vi "calc T and P.vi"(7 "DAQ state cluster in in":T1={"DAQ state"=enum."Global comm", "device"="", "start (ms)"=0, "error"={"status"=FALSE, "code"=0, "source"=""}, "T cont"={"exec"={"T mode"=enum."Setting up", "man power"=0.0, "log"=FALSE}, "T status"={"Temp"=0.0, "Power"=0.0}, "utility"={"meas index"=0, "wait (ms)"=0, "H Vmax"=8.5, "power out"=5.0, "heat volt out"=0.0, "heat volt in"=0.0, "therm volt"=0.0, "t T P hist"=[]}}} {"T cont"."utility"."therm volt" format="%_6g"; "T cont"."utility"."heat volt in" format="%_6g"; "T cont"."utility"."heat volt out" format="%_6g"; "T cont"."utility"."power out" format="%_6g"; "T cont"."utility"."H Vmax" format="%_6g"; "T cont"."exec"."man power" format="%_6g"; "T cont"."T status"."Power" format="%_6g"; "T cont"."T status"."Temp" format="%_6g"}) -> (8 "DAQ state cluster out":T1={"DAQ state"=enum."Global comm", "device"="", "start (ms)"=0, "error"={"status"=FALSE, "code"=0, "source"=""}, "T cont"={"exec"={"T mode"=enum."Setting up", "man power"=0.0, "log"=FALSE}, "T status"={"Temp"=0.0, "Power"=0.0}, "utility"={"meas index"=0, "wait (ms)"=0, "H Vmax"=8.5, "power out"=5.0, "heat volt out"=0.0, "heat volt in"=0.0, "therm volt"=0.0, "t T P hist"=[]}}} {"T cont"."utility"."therm volt" format="%_6g"; "T cont"."utility"."heat volt in" format="%_6g"; "T cont"."utility"."heat volt out" format="%_6g"; "T cont"."utility"."power out" format="%_6g"; "T cont"."utility"."H Vmax" format="%_6g"; "T cont"."exec"."man power" format="%_6g"; "T cont"."T status"."Power" format="%_6g"; "T cont"."T status"."Temp" format="%_6g"})   [LabVIEW 2019]
doc: "This subVI is a component of the meas T and P state of the DAQ state machine in the bug experiment.\n\nThis subVI calculates the current time, the bug temerature, and the bug heater power from the raw voltage measurements and saves the data to arunning array for graphing.\n\nIt records the history of the time, temperature, and power.\nIt also logs the temp control parameters is logging is active.\n\nPaul K Dixon\nP3600\nCSUSB Physics"
uses:
  typedefs/DAQ T state cluster.ctl
  typedefs/DAQ T state enum.ctl
  typedefs/temp cont cluster.ctl
  typedefs/temp exec cluster.ctl
  typedefs/temp mode enum.ctl
  typedefs/temp indicator.ctl
  typedefs/temp cont utility.ctl
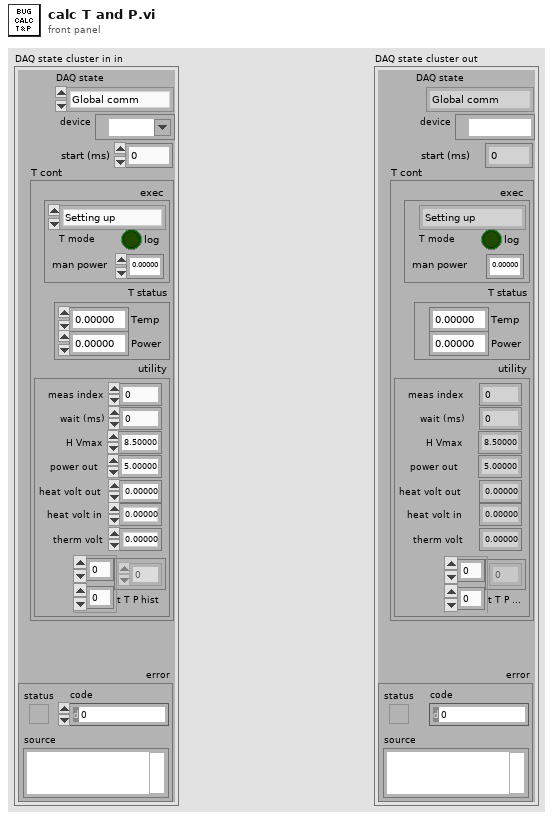
[diagram p1: front panel]
types:
  T1 = typedef "DAQ T state cluster.ctl" = cluster{"DAQ state":T2, "device":tag, "start (ms)":i32, "error":errorcluster, "T cont":T3}
  T2 = typedef "DAQ T state enum.ctl" = enum16{"Global comm", "Meas T & P", "Man Power set", "Output Power", "Wait", "Exit"}
  T3 = typedef "temp cont cluster.ctl" = cluster{"exec":T4, "T status":T6, "utility":T7}
  T4 = typedef "temp exec cluster.ctl" = cluster{"T mode":T5, "man power":dbl, "log":bool}
  T5 = typedef "temp mode enum.ctl" = enum16{"Setting up", "Listening to exec", "Exit"}
  T6 = typedef "temp indicator.ctl" = cluster{"Temp":dbl, "Power":dbl}
  T7 = typedef "temp cont utility.ctl" = cluster{"meas index":i32, "wait (ms)":i32, "H Vmax":dbl, "power out":dbl, "heat volt out":dbl, "heat volt in":dbl, "therm volt":dbl, "t T P hist":dbl[][]}
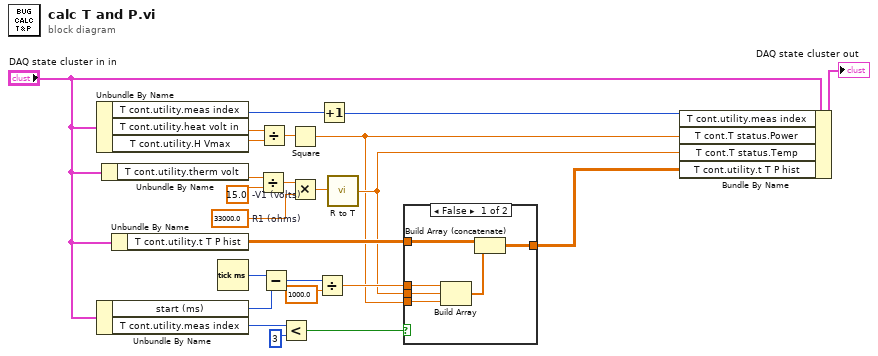
[diagram p0: block diagram]
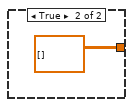
[diagram p2: hidden frame]
diagram:
  w19 = 15.0  # -V1 (volts)
  w17 = 33000.0  # R1 (ohms)
  n1 = Unbundle By Name("DAQ state cluster in in") -> ("T cont.utility.meas index"=w6:i32, "T cont.utility.heat volt in"=w23:dbl, "T cont.utility.H Vmax"=w22:dbl)
  n2 = Unbundle By Name("DAQ state cluster in in") -> ("start (ms)"=w13:i32, "T cont.utility.meas index"=w3:i32)
  n3 = Unbundle By Name("DAQ state cluster in in") -> ("T cont.utility.therm volt"=w20:dbl)
  n4 = Unbundle By Name("DAQ state cluster in in") -> ("T cont.utility.t T P hist"=w15:dbl[][])
  n5 = Tick Count (ms)() -> (millisecond timer value=w14:u32)
  n6 = Divide(x=w20, y=w19) -> (x/y=w18:dbl)
  n7 = Divide(x=w23, y=w22) -> (x/y=w21:dbl)
  n8 = Subtract(x=w14, y=w13) -> (x-y=w12:u32)
  n9 = Less?(x=w3, y=3) -> (x < y?=w1:bool)
  n10 = Square(x=w21) -> (x^2=w7:dbl)
  n11 = Multiply(x=w18, y=w17) -> (x*y=w16:dbl)
  n12 = Divide(x=w12, y=1000.0) -> (x/y=w9:dbl)
  n13 = Increment(x=w6) -> (x+1=w5:i32)
  n14 = call "R to T.vi"("Resistance (Ohm)"=w16) -> ("Temp (deg C)"=w8:dbl)  [unwired: 13 in, 1 out]
  n15 = case shown="False" w1 {
    tunnel: w15 -> [w30 _]
    tunnel: w9 -> [w29 _]
    tunnel: w8 -> [w28 _]
    tunnel: w7 -> [w26 _]
    tunnel: [w25 dbl[][] []] -> w4
    frame False {
      n16 = Build Array(w29, w28, w26) -> (w27:dbl[])
      n17 = Build Array (concatenate)(w30, w27) -> (w25:dbl[][])
    }
    frame True {
    }
  }
  n18 = Bundle By Name(cluster="DAQ state cluster in in", "T cont.utility.meas index"=w5, "T cont.T status.Power"=w7, "T cont.T status.Temp"=w8, "T cont.utility.t T P hist"=w4) -> (→"DAQ state cluster out":T1)
